vi "Convert to Eng, P and T.vi"(0 "Pmin (Pa)":sgl format="%#_13g", 1 "P word":string, 2 "OutputMin (counts)":sgl format="%#_13g", 3 "Poffset (Pa)":sgl format="%#_13g", 4 "T word":string, 5 "(Pmax - Pmin) / (OutputMax - OutputMin) (Pa/count)":sgl format="%#_13g") -> (6 "P (Pa)":sgl, 7 "T (degC)":sgl, 8 "Status bit":u8)   [LabVIEW 2015]
panel:
  # "0: valid data\n1: cmd mode\n2: stale data\n3: diag mode"
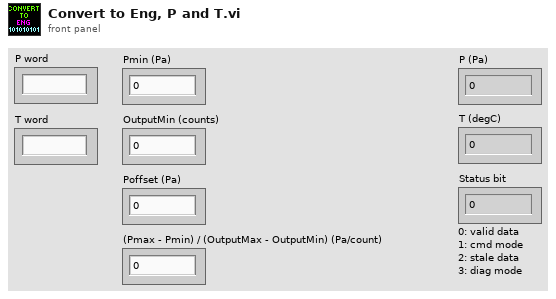
[diagram p1: front panel]
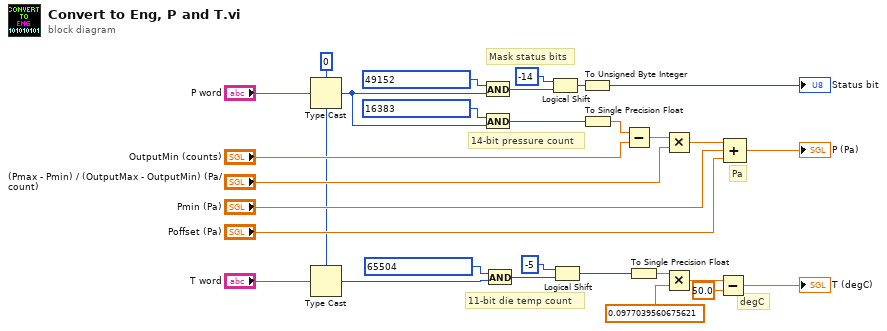
[diagram p0: block diagram]
diagram:
  w3 = u16 0
  # "degC"
  # "11-bit die temp count"
  # "Pa"
  # "14-bit pressure count"
  # "Mask status bits"
  n1 = Type Cast(type=w3, x="P word") -> (*(type *) &x=w1:u16)
  n2 = Type Cast(type=w3, x="T word") -> (*(type *) &x=w2:u16)
  n3 = And(x=u16 49152, y=w1) -> (x .and. y?=w19:u16)
  n4 = And(x=u16 16383, y=w1) -> (x .and. y?=w25:u16)
  n5 = And(x=u16 65504, y=w2) -> (x .and. y?=w13:u16)
  n6 = Logical Shift(y=i16 -14, x=w19) -> (x << y=w21:u16)
  n7 = Logical Shift(y=i16 -5, x=w13) -> (x << y=w7:u16)
  n8 = To Unsigned Byte Integer(number=w21) -> (unsigned 8bit integer=→"Status bit":u8)
  n9 = To Single Precision Float(number=w25) -> (single precision float=w26:sgl)
  n10 = Subtract(x=w26, y="OutputMin (counts)") -> (x-y=w27:sgl)
  n11 = To Single Precision Float(number=w7) -> (single precision float=w8:sgl)
  n12 = Multiply(x=w27, y="(Pmax - Pmin) / (OutputMax - OutputMin) (Pa/count)") -> (x*y=w15:sgl)
  n13 = Multiply(x=w8, y=sgl 0.097703956) -> (x*y=w10:sgl)
  n14 = Subtract(x=w10, y=sgl 50.0) -> (x-y=→"T (degC)":sgl)
  n15 = Compound Arithmetic op=ADD(w15, "Pmin (Pa)", "Poffset (Pa)") -> (→"P (Pa)":sgl)
